vi "Count up to 17575 with 3 Characters.vi"(1 "Numeric Control":i32) -> (0 "string":string)   [LabVIEW 2015]
panel:
  out "NumberOfCharacters":i32
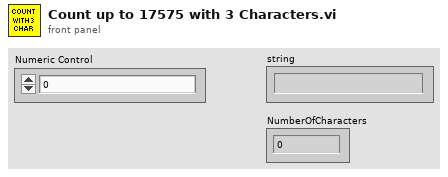
[diagram p1: front panel]
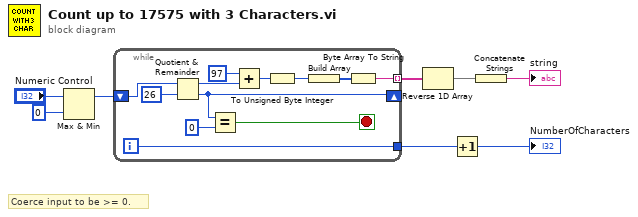
[diagram p0: block diagram]
diagram:
  # "Coerce input to be >= 0."
  n1 = Max & Min(x="Numeric Control", y=0) -> (max(x,y)=w4:i32)  [unwired: 1 out]
  n2 = while {
    shift-right: [w11] -> _
    shift-left: w4 -> [w12]
    tunnel: [w17] -> w8 mode=indexing
    tunnel: [w16] -> w2
    i -> [w16]
    stop <- w14 stop-if-true
    n3 = Quotient & Remainder(x=w12, y=26) -> (x-y*floor(x/y)=w13:i32, floor(x/y)=w11:i32)
    n4 = Equal?(x=w11, y=0) -> (x = y?=w14:bool)
    n5 = Add(x=97, y=w13) -> (x+y=w10:i32)
    n6 = To Unsigned Byte Integer(number=w10) -> (unsigned 8bit integer=w9:u8)
    n7 = Build Array(w9) -> (w19:u8[])
    n8 = Byte Array To String(unsigned byte array=w19) -> (string=w17:string)
  }
  n9 = Reverse 1D Array(array=w8) -> (reversed array=w7:string[])
  n10 = Increment(x=w2) -> (x+1=→"NumberOfCharacters":i32)
  n11 = Concatenate Strings(w7) -> (→"string":string)
